vi "Ejercicio 3.2.vi"() -> ()   [LabVIEW 2020]
panel:
  out "Gráfico de seno y coseno":cluster{cluster{dbl, dbl}[]}[](graph) caption="XY Graph"
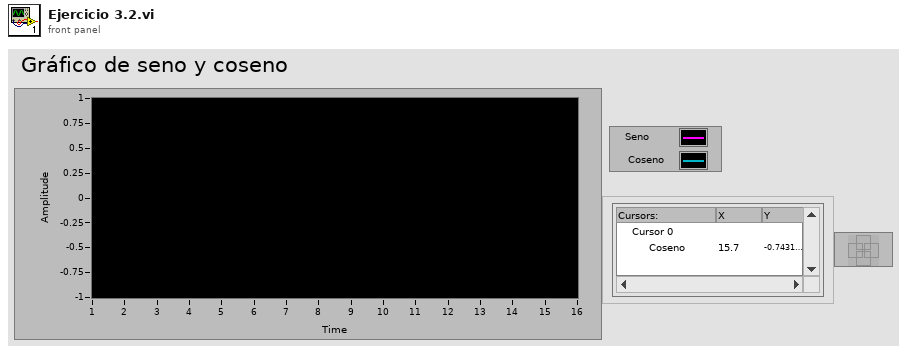
[diagram p1: front panel]
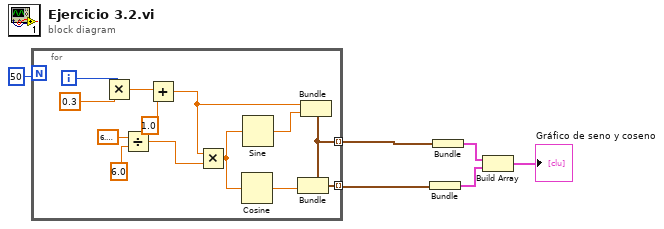
[diagram p0: block diagram]
diagram:
  n1 = for {
    N: 50 -> [_]
    tunnel: [w7] -> w5 mode=indexing
    tunnel: [w13] -> w4 mode=indexing
    i -> [w15]
    n2 = Multiply(x=w15, y=0.3) -> (x*y=w19:dbl)
    n3 = Divide(x=6.283185307179586, y=6.0) -> (x/y=w18:dbl)
    n4 = Add(x=w19, y=1.0) -> (x+y=w11:dbl)
    n5 = Multiply(x=w11, y=w18) -> (x*y=w12:dbl)
    n6 = Cosine(x=w12) -> (cos(x)=w14:dbl)
    n7 = Sine(x=w12) -> (sin(x)=w16:dbl)
    n8 = Bundle(w11, w16) -> (w7:cluster{dbl, dbl})  [unwired: 1 in]
    n9 = Bundle(cluster=w7, w14) -> (w13:cluster{dbl, dbl})  [unwired: 1 in]
  }
  n10 = Bundle(w4) -> (w2:cluster{cluster{dbl, dbl}[]})  [unwired: 1 in]
  n11 = Bundle(w5) -> (w3:cluster{cluster{dbl, dbl}[]})  [unwired: 1 in]
  n12 = Build Array(w3, w2) -> (→"Gráfico de seno y coseno":cluster{cluster{dbl, dbl}[]}[])
